vi "hydraharp_insert_into_moving_buffer_dbl.vi"(8 "elements_in_buffer":i32, 9 "buffer_size":i32, 10 "new_data":dbl[](array[numeric]), 11 "buffer":dbl[](array[numeric])) -> (0 "elements_in_new_buffer":i32, 1 "buffer_size 2":i32, 3 "new_buffer":dbl[](array[numeric]))   [LabVIEW 2015, in "hydraharp.lvclass"]
uses:
  hydraharp.lvclass
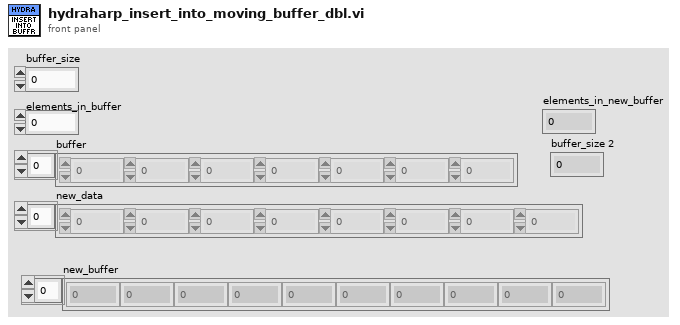
[diagram p1: front panel]
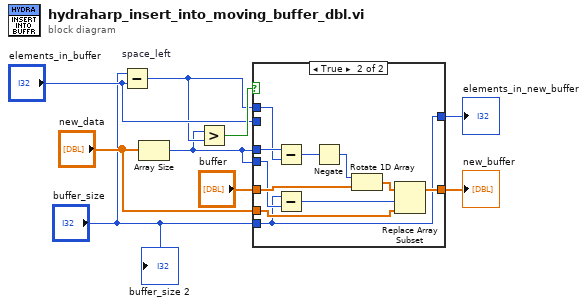
[diagram p0: block diagram]
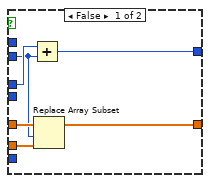
[diagram p2: hidden frame]
diagram:
  n1 = Subtract "space_left"(x="buffer_size", y="elements_in_buffer") -> (x-y=w4:i32)
  n2 = Array Size(array="new_data") -> (size(s)=w2:i32)
  n3 = Greater?(x=w2, y=w4) -> (0:w9:bool)
  n4 = case shown="True" w9 {
    tunnel: "buffer" -> [w15 w26]
    tunnel: "elements_in_buffer" -> [w11 _]
    tunnel: "new_data" -> [w14 w20]
    tunnel: [w13 w17] -> w5
    tunnel: w2 -> [w12 w25]
    tunnel: w4 -> [_ w24]
    tunnel: "buffer_size" -> [_ w16]
    tunnel: w2 -> [_ w19]
    tunnel: [w10 w16] -> w1
    frame False {
      n5 = Add(x=w12, y=w11) -> (x+y=w10:i32)
      n6 = Replace Array Subset(array=w15, new element=w14, index=w11) -> (w13:dbl[])
    }
    frame True {
      n7 = Subtract(x=w25, y=w24) -> (x-y=w23:i32)
      n8 = Subtract(x=w16, y=w19) -> (x-y=w18:i32)
      n9 = Negate(x=w23) -> (-x=w22:i32)
      n10 = Rotate 1D Array(1:w26, 2:w22) -> (0:w21:dbl[])
      n11 = Replace Array Subset(array=w21, new element=w20, index=w18) -> (w17:dbl[])
    }
  }
  "new_buffer" <- w5
  "elements_in_new_buffer" <- w1
  "buffer_size 2" <- "buffer_size"
